vi "kepcoScanStandAlone.vi"(4 "abort":bool, 5 "halt":bool, 6 "invertInOddnOfTrack":bool, 8 "Go":bool, 9 "nOfScanRegions":i32, 10 "waitForKepco(25nsTicks)":u16, 11 "waitForDmm(25nsTicks)":u32) -> (0 "timeoutDAC":bool)   [LabVIEW 2014]
uses:
  <vilib>/rvi/Emulation/niFpgaGetClockAttributes.vi
  <vilib>/rvi/Emulation/niFpgaSctlEmulationGetInTimedLoop.vi
  <vilib>/rvi/Emulation/niFpgaEmulationReportErrorSimple.vi
  Sequencer/sequencerGlobVars.vi
  <vilib>/rvi/Emulation/niFpgaProcessEmulError.vi
  DAC/Code/FPGA SPI_Globals.vi
  <vilib>/rvi/Emulation/niFpgaCriticalErrorInLSC.vi
panel:
  in  "waitAfterReset(25nsTicks)":u16
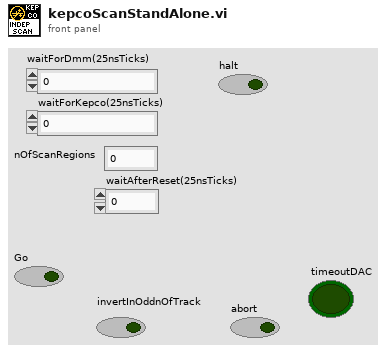
[diagram p1: front panel]
types:
  T1 = cluster{"SCLK":refnum<k21>, "CS":refnum<k21>, "MOSI":refnum<k21>, "MISO":refnum<k21>}
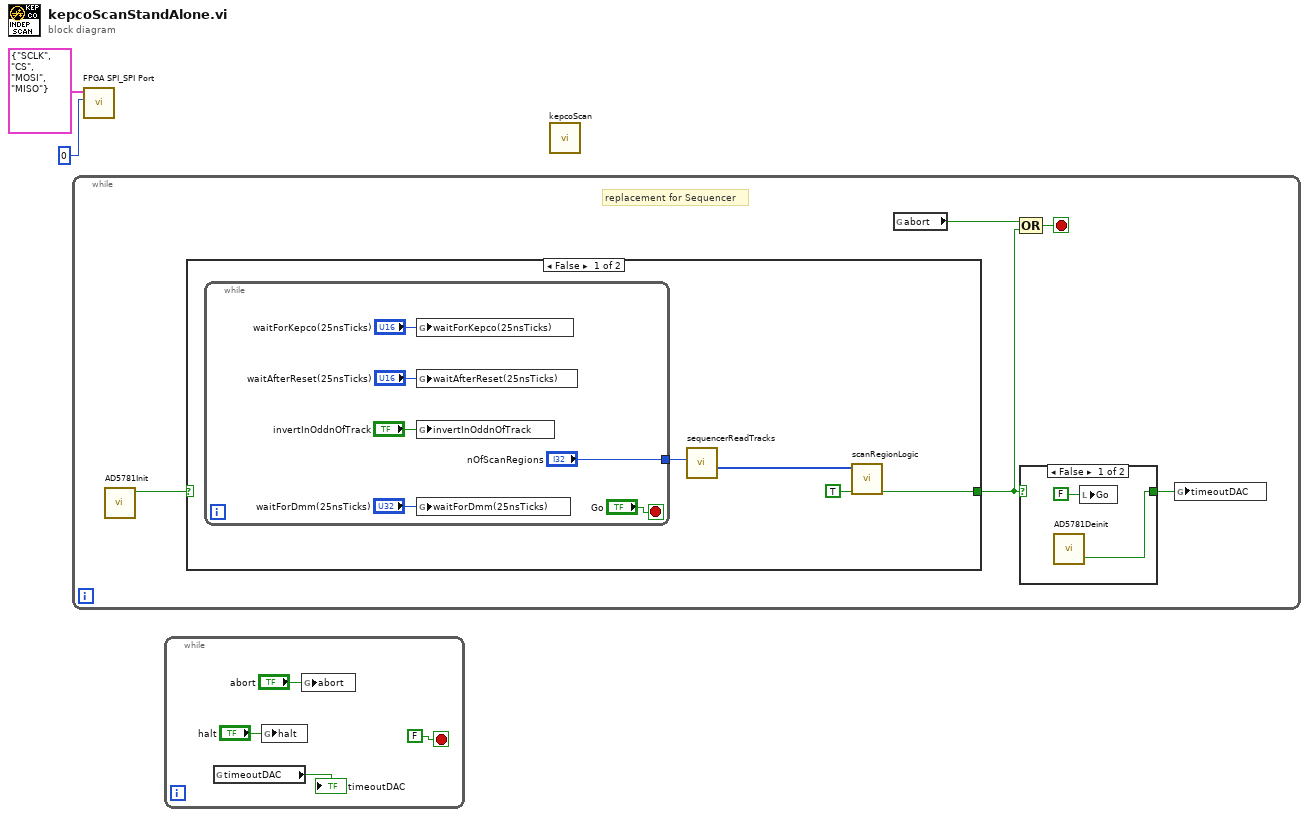
[diagram p0: block diagram]
diagram:
  n1 = while {
    stop <- w4 stop-if-true
    # "replacement for Sequencer"
    n2 = call "AD5781Init.vi"() -> ("timeOut"=w7:bool)  [unwired: 11 in]
    n3 = case shown="False" w7 {
      selector: w7 -> [_ w21]
      tunnel: [w11 w21] -> w3
      frame False {
        n4 = while {
          tunnel: ["nOfScanRegions"] -> w14
          stop <- "Go" stop-if-true
          n5 = global write "FPGA SPI_Globals.vi" "waitForKepco(25nsTicks)"("waitForKepco(25nsTicks)") -> ()
          n6 = global write "FPGA SPI_Globals.vi" "waitAfterReset(25nsTicks)"("waitAfterReset(25nsTicks)") -> ()
          n7 = global write "FPGA SPI_Globals.vi" "invertInOddnOfTrack"("invertInOddnOfTrack") -> ()
          n8 = global write "FPGA SPI_Globals.vi" "waitForDmm(25nsTicks)"("waitForDmm(25nsTicks)") -> ()
        }
        n9 = call "sequencerReadTracks.vi"("nOfScanRegions"=w14) -> ("arrayOfTracks"=w13:i32[])  [unwired: 10 in]
        n10 = call "scanRegionLogic.vi"("kepcoScan"=TRUE, "Array of Tracks"=w13) -> ("Error"=w11:bool)  [unwired: 9 in]
      }
      frame True {
      }
    }
    n11 = global read "sequencerGlobVars.vi" "abort"() -> (w5:bool)
    n12 = Compound Arithmetic op=OR(w5, w3) -> (w4:bool)
    n13 = case shown="False" w3 {
      selector: w3 -> [_ w10]
      tunnel: [w9 w10] -> w6
      frame False {
        n14 = call "AD5781Deinit.vi"() -> ("timedOut"=w9:bool)  [unwired: 3 in]
        n15 = local write "Go"(FALSE ("Go")) -> ()
      }
      frame True {
      }
    }
    n16 = global write "FPGA SPI_Globals.vi" "timeoutDAC"(w6) -> ()
  }
  n17 = call "FPGA SPI_SPI Port.vi"("Port"=i8 0, "FPGA IO"=T1 {"SCLK"="SCLK", "CS"="CS", "MOSI"="MOSI", "MISO"="MISO"}) -> ()  [unwired: 10 in]
  n18 = while {
    stop <- FALSE stop-if-true
    n19 = global read "FPGA SPI_Globals.vi" "timeoutDAC"() -> (→"timeoutDAC":bool)
    n20 = global write "sequencerGlobVars.vi" "halt"("halt") -> ()
    n21 = global write "sequencerGlobVars.vi" "abort"("abort") -> ()
  }
  n22 = call "kepcoScan.vi"() -> ()  [unwired: 12 in]
